vi "SW_Save_Cluster_from_String.vi"(0 "Data String in":string, 2 "Settings cluster in":T1 {"Calibration parameters"."True frame time, s" format="%.10g"; "Calibration parameters"."Disp. calibration info"."Speed, µl per ms" format="%.3g"; "Calibration parameters"."True FPS" format="%.10g"; "Calibration parameters"."Timing calibration sw/hw" format="%.10g"; "Conditions presets array"."Specifier(s)"."Validity criteria(s)"."Validity value" min=0.0 step=0.1 format="%.2g"; "Conditions presets array"."Specifier(s)"."Value" step=1.0 format="%#.2g"; "Recording and saving"."Data post-processing"."Order" min=3 max=11 step=2; "Recording and saving"."Data post-processing"."Length" min=5 max=301 step=2; "Geometry"."Cage type" items=["Round", "Square", "Donut-maze", "T-maze", "Sociability maze", ""]}, 3 "error in (no error)":errorcluster) -> (5 "Settings cluster out":T1 {"Calibration parameters"."True frame time, s" format="%.10g"; "Calibration parameters"."Disp. calibration info"."Speed, µl per ms" format="%.3g"; "Calibration parameters"."True FPS" format="%.10g"; "Calibration parameters"."Timing calibration sw/hw" format="%.10g"; "Conditions presets array"."Specifier(s)"."Validity criteria(s)"."Validity value" min=0.0 step=0.1 format="%.2g"; "Conditions presets array"."Specifier(s)"."Value" step=1.0 format="%#.2g"; "Recording and saving"."Data post-processing"."Order" min=3 max=11 step=2; "Recording and saving"."Data post-processing"."Length" min=5 max=301 step=2; "Geometry"."Cage type" items=["Round", "Square", "Donut-maze", "T-maze", "Sociability maze", ""]}, 7 "error out":errorcluster)   [LabVIEW 2018, in "Tracker.lvlib"]
uses:
  Tracker.lvlib
  Controls/CTL_Settings_cluster.ctl
  Controls/CTL_Histogram_parameters.ctl
  Controls/CTL_Filter_selector.ctl
  Controls/CTL_Acquisition_speed_selector.ctl
  Controls/CTL_Segmented_plot_parameters_2.ctl
  Libraries/Cage Diagram/Typedefs/CTL_Cage_type.ctl
  Controls/CTL_Cage_all_segmentation_params_set.ctl
  Controls/CTL_IO_params_cluster.ctl
  Controls/CTL_Conditions_Array.ctl
  Controls/CTL_Conditions_Cluster.ctl
  Controls/CTL_Condition_type.ctl
  Controls/CTL_Comparison_type.ctl
  Controls/CTL_Validity_check_criteria.ctl
  Controls/CTL_Response_info.ctl
  Controls/CTL_Condition_response_type.ctl
  Controls/CTL_Reponse_port_info.ctl
  Controls/CTL_Calibration_parameters.ctl
  Controls/CTL_Dispenser_calibration_info.ctl
  Common_Resources.lvlib
  Libraries/Cage Diagram/Cage Diagram.lvlib
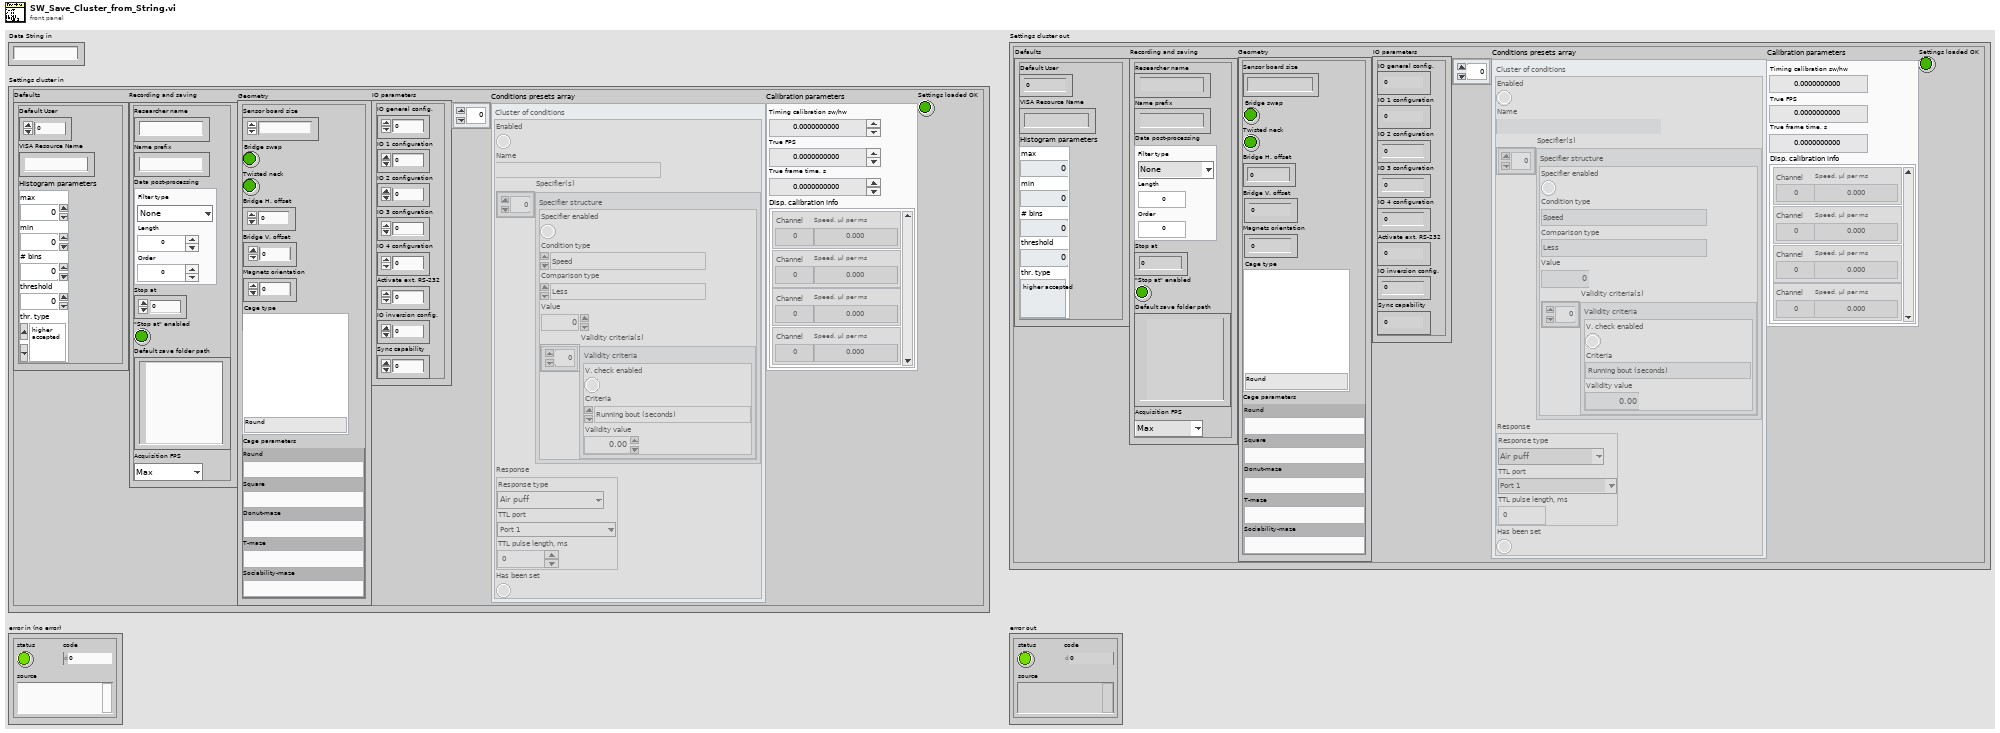
[diagram p1: front panel]
types:
  T1 = typedef "Common_Resources.lvlib/CTL_Settings_cluster.ctl" = cluster{"Defaults":cluster{"Default User":dbl, "VISA Resource Name ":string, "Histogram parameters":T2}, "Recording and saving":cluster{"Researcher name":string, "Name prefix":string, "Data post-processing":T3, "Stop at":dbl, "\"Stop at\" enabled":bool, "Default save folder path":path, "Acquisition FPS":T4}, "Geometry":T5, "IO parameters":T8, "Conditions presets array":T9, "Calibration parameters":T17, "Settings loaded OK":bool}
  T2 = typedef "Common_Resources.lvlib/CTL_Histogram_parameters.ctl" = cluster{"max":dbl, "min":dbl, "# bins":i32, "threshold":dbl, "thr. type":enum16{"higher accepted", "lower accepted"}}
  T3 = typedef "Common_Resources.lvlib/CTL_Filter_selector.ctl" = cluster{"Filter type":enum16{"None", "Savitzky-Golay"}, "Length":i32, "Order":i32}
  T4 = typedef "Common_Resources.lvlib/CTL_Acquisition_speed_selector.ctl" = enum16{"Max", "Optimal", "Eco"}
  T5 = typedef "Common_Resources.lvlib/CTL_Segmented_plot_parameters_2.ctl" = cluster{"Sensor board size":enum16{"", "Large"}, "Bridge swap":bool, "Twisted neck":bool, "Bridge H. offset":sgl, "Bridge V. offset":sgl, "Magnets orientation":sgl, "Cage type":T6, "Cage parameters":T7}
  T6 = typedef "Cage Diagram.lvlib/CTL_Cage_type.ctl" = u16
  T7 = typedef "Common_Resources.lvlib/CTL_Cage_all_segmentation_params_set.ctl" = cluster{"Round":variant, "Square":variant, "Donut-maze":variant, "T-maze":variant, "Sociability-maze":variant}
  T8 = typedef "Common_Resources.lvlib/CTL_IO_params_cluster.ctl" = cluster{"IO general config.":u16, "IO 1 configuration":u16, "IO 2 configuration":u16, "IO 3 configuration":u16, "IO 4 configuration":u16, "Activate ext. RS-232":u16, "IO inversion config.":u16, "Sync capability":u8}
  T9 = typedef "Common_Resources.lvlib/CTL_Conditions_Array.ctl" = T10[]
  T10 = typedef "Common_Resources.lvlib/CTL_Conditions_Cluster.ctl" = cluster{"Enabled":bool, "Name":string, "Specifier(s)":cluster{"Specifier enabled":bool, "Condition type":T11, "Comparison type":T12, "Value":dbl, "Validity criteria(s)":cluster{"V. check enabled":bool, "Criteria":T13, "Validity value":dbl}[]}[], "Response":T14, "Has been set":bool}
  T11 = typedef "Common_Resources.lvlib/CTL_Condition_type.ctl" = enum16{"Speed", "Zone", "Angle to wall"}
  T12 = typedef "Common_Resources.lvlib/CTL_Comparison_type.ctl" = enum16{"Less", "Less or Equal", "Equal", "Greater or Equal", "Greater", "Not Equal"}
  T13 = typedef "Common_Resources.lvlib/CTL_Validity_check_criteria.ctl" = enum16{"Running bout (seconds)", "Running bout (meters)"}
  T14 = typedef "Common_Resources.lvlib/CTL_Response_info.ctl" = cluster{"Response type":T15, "TTL port":T16, "TTL pulse length, ms":dbl}
  T15 = typedef "Common_Resources.lvlib/CTL_Condition_response_type.ctl" = enum16{"None", "Air puff", "Liquid reward", "TTL pulse", "TTL pulse (ubr)", "TTL signal"}
  T16 = typedef "Common_Resources.lvlib/CTL_Reponse_port_info.ctl" = enum16{"Port 1", "Port 2", "Port 3", "Port 4"}
  T17 = typedef "Common_Resources.lvlib/CTL_Calibration_parameters.ctl" = cluster{"Timing calibration sw/hw":dbl, "True FPS":dbl, "True frame time, s":dbl, "Disp. calibration info":T18}
  T18 = typedef "Common_Resources.lvlib/CTL_Dispenser_calibration_info.ctl" = cluster{"Channel":u8, "Speed, µl per ms":dbl}[]
  T19 = cluster{"Default User":dbl, "VISA Resource Name ":string, "Histogram parameters":T2}
  T20 = cluster{"Researcher name":string, "Name prefix":string, "Data post-processing":T3, "Stop at":dbl, "\"Stop at\" enabled":bool, "Default save folder path":path, "Acquisition FPS":T4}
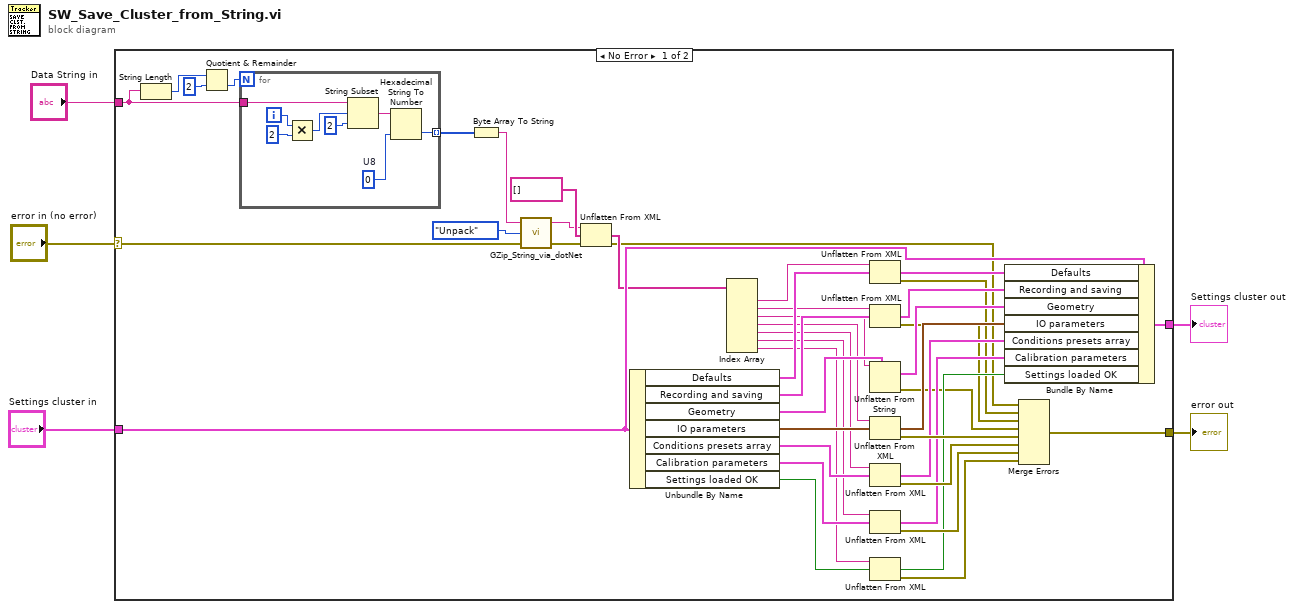
[diagram p0: block diagram]
diagram:
  n1 = case shown="No Error" "error in (no error)" {
    selector: "error in (no error)" -> [w6 w58]
    tunnel: "Settings cluster in" -> [w42 w59]
    tunnel: [w26 w59] -> w4
    tunnel: [w23 w58] -> w3
    tunnel: "Data String in" -> [w8 _]
    frame No Error {
      n2 = String Length(string=w8) -> (length=w12:i32)
      n3 = Quotient & Remainder(x=w12, y=2) -> (floor(x/y)=w10:i32)  [unwired: 1 out]
      n4 = for {
        N: w10 -> [_]
        tunnel: w8 -> [w57]
        tunnel: [w50] -> w9 mode=indexing
        i -> [w55]
        w51 = u8 0  # U8
        n5 = Multiply(x=w55, y=2) -> (x*y=w54:i32)
        n6 = String Subset(string=w57, offset (0)=w54, length (rest)=2 ("length (rest)")) -> (substring=w52:string)
        n7 = Hexadecimal String To Number(string=w52, default (0uL)=w51) -> (number=w50:u8)  [unwired: 1 in, 1 out]
      }
      n8 = Byte Array To String(unsigned byte array=w9) -> (string=w7:string)
      n9 = call "GZip_String_via_dotNet.vi"("error in (no error)"=w6, "Action"=enum16{"Pack", "Unpack"}."Unpack", "String Input"=w7) -> ("error out"=w13:errorcluster, "String Output (GZipped/UnGZipped)"=w15:string)  [unwired: 1 out]
      n10 = Unflatten From XML(xml string=w15, type=string[] [], error in (no error)=w13) -> (value=w17:string[], error out=w16:errorcluster)
      n11 = Unbundle By Name(w42) -> ("Defaults"=w43:T19, "Recording and saving"=w44:T20, "Geometry"=w45:T5, "IO parameters"=w46:T8, "Conditions presets array"=w47:T9, "Calibration parameters"=w48:T17, "Settings loaded OK"=w49:bool)
      n12 = Index Array(array=w17) -> (element #1=w19:string, element #2=w20:string, element #3=w27:string, element #4=w38:string, element #5=w39:string, element #6=w40:string, element #7=w41:string)  [unwired: 7 in]
      n13 = Unflatten From XML(xml string=w19, type=w43) -> (value=w24:T19, error out=w21:errorcluster)  [unwired: 1 in]
      n14 = Unflatten From XML(xml string=w20, type=w44) -> (value=w25:T20, error out=w22:errorcluster)  [unwired: 1 in]
      n15 = Unflatten From String(type=w45, binary string=w27) -> (value=w28:T5, error out=w29:errorcluster)  [unwired: 3 in, 1 out]
      n16 = Unflatten From XML(xml string=w38, type=w46) -> (value=w30:T8, error out=w34:errorcluster)  [unwired: 1 in]
      n17 = Unflatten From XML(xml string=w39, type=w47) -> (value=w31:T9, error out=w35:errorcluster)  [unwired: 1 in]
      n18 = Unflatten From XML(xml string=w40, type=w48) -> (value=w32:T17, error out=w36:errorcluster)  [unwired: 1 in]
      n19 = Unflatten From XML(xml string=w41, type=w49) -> (value=w33:bool, error out=w37:errorcluster)  [unwired: 1 in]
      n20 = Bundle By Name(cluster=w42, "Defaults"=w24, "Recording and saving"=w25, "Geometry"=w28, "IO parameters"=w30, "Conditions presets array"=w31, "Calibration parameters"=w32, "Settings loaded OK"=w33) -> (w26:T1)
      n21 = Merge Errors(w16, w21, w22, w29, w34, w35, w36, w37) -> (w23:errorcluster)
    }
    frame Error {
    }
  }
  "Settings cluster out" <- w4
  "error out" <- w3
